vi "HP33120Aoutsine0516.VI"() -> ()   [LabVIEW 2017]
uses:
  <vilib>/Analysis/NI_AALBase.lvlib
panel:
  in  "幅值":dbl
  in  "频率":dbl
  in  "相位":dbl caption="相位（度）" format="%0.2f"
  in  "采样":i32=128
  out "波形图":waveform(dbl)(graph)
  in  "串口参数设置":enum32{"常用设置", "不常用的"}(tab)
  in  "VISA resource name":refnum<visa-resource-name>="COM1" caption="端口号"
  in  "baud rate":u32=9600 caption="波特率"
  in  "parity":u16(ring) caption="奇偶校验" items=["None", "Odd", "Even", "Mark", "Space"]
  in  "stop bits":u16(ring)=10 caption="停止位" items=["1.0"=10, "1.5"=15, "2.0"=20]
  in  "data bits":u16=8 caption="数据位" min=5 max=8 step=1
  in  "flow control":u16(ring) caption="流量控制" items=["None"=0, "XON/XOFF"=1, "RTS/CTS"=2, "DTR/DSR"=4]
  in  "termination char\n(0xA = '\\n' = LF)":u8=10 caption="EOL字串-LF" format="%.0x"
  in  "Input buffer size":u32=4096 caption="输入缓冲区大小"
  in  "XOFF Character":u8=19 format="%.0x"
  in  "XON Character":u8=17 format="%.0x"
  in  "timeout (ms)":u32=10000
  # "输出波形信息"
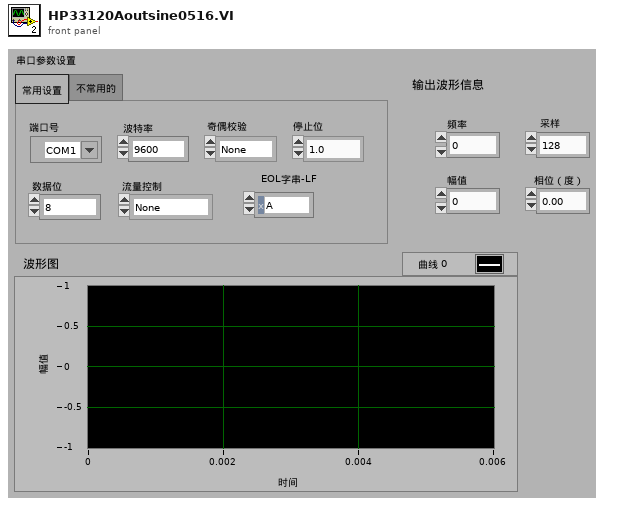
[diagram p1: front panel]
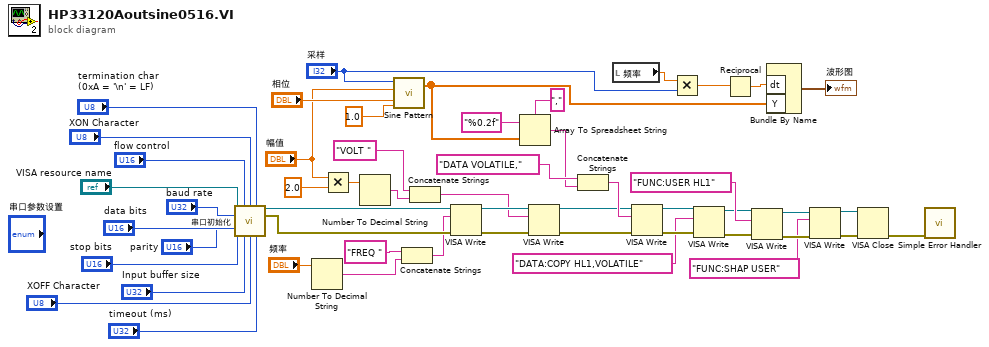
[diagram p0: block diagram]
diagram:
  n1 = call "串口初始化.vi"("VISA resource name"="VISA resource name", "flow control"="flow control", "XON Character"="XON Character", "termination char\n(0xA = '\\n' = LF)"="termination char\n(0xA = '\\n' = LF)", "baud rate"="baud rate", "data bits"="data bits", "parity"="parity", "stop bits"="stop bits", "Input buffer size"="Input buffer size", "XOFF Character"="XOFF Character", "timeout (ms)"="timeout (ms)") -> ("VISA resource name out"=w37:refnum<visa-resource-name>, "错误输出"=w36:errorcluster)  [unwired: 3 in]
  n2 = Number To Decimal String(number="频率") -> (decimal integer string=w17:string)  [unwired: 1 in]
  n3 = Multiply(x="幅值", y=2.0) -> (x*y=w1:dbl)
  n4 = Number To Decimal String(number=w1) -> (decimal integer string=w14:string)  [unwired: 1 in]
  n5 = call <vilib>:"Sine Pattern.vi"("cycles"=1.0, "phase(degrees)"="相位", "amplitude"="幅值", "samples"="采样") -> ("Sinusoidal Pattern"=w10:dbl[])  [unwired: 1 out]
  n6 = Concatenate Strings("FREQ " ("写入缓冲区"), w17) -> (w16:string)
  n7 = Concatenate Strings("VOLT " ("写入缓冲区"), w14) -> (w5:string)
  n8 = VISA Write(VISA resource name=w37, write buffer=w16, error in (no error)=w36) -> (VISA resource name out=w35:refnum<visa-resource-name>, error out=w34:errorcluster)  [unwired: 1 out]
  n9 = Array To Spreadsheet String(delimiter (Tab)="," ("分隔符(Tab)"), array=w10, 3:"%0.2f" ("格式字符串")) -> (spreadsheet string=w19:string)
  n10 = VISA Write(VISA resource name=w35, write buffer=w5, error in (no error)=w34) -> (VISA resource name out=w33:refnum<visa-resource-name>, error out=w32:errorcluster)  [unwired: 1 out]
  n11 = Concatenate Strings("DATA VOLATILE," ("写入缓冲区"), w19) -> (w38:string)
  n12 = local read "频率"() -> (w9:dbl)
  n13 = VISA Write(VISA resource name=w33, write buffer=w38, error in (no error)=w32) -> (VISA resource name out=w22:refnum<visa-resource-name>, error out=w21:errorcluster)  [unwired: 1 out]
  n14 = Multiply(x=w9, y="采样") -> (x*y=w6:dbl)
  n15 = VISA Write(VISA resource name=w22, write buffer="DATA:COPY HL1,VOLATILE" ("写入缓冲区"), error in (no error)=w21) -> (VISA resource name out=w30:refnum<visa-resource-name>, error out=w29:errorcluster)  [unwired: 1 out]
  n16 = Reciprocal(x=w6) -> (1/x=w8:dbl)
  n17 = VISA Write(VISA resource name=w30, write buffer="FUNC:USER HL1" ("写入缓冲区"), error in (no error)=w29) -> (VISA resource name out=w28:refnum<visa-resource-name>, error out=w27:errorcluster)  [unwired: 1 out]
  n18 = Bundle By Name("dt"=w8, "Y"=w10) -> (→"波形图":waveform(dbl))  [unwired: 1 in]
  n19 = VISA Write(VISA resource name=w28, write buffer="FUNC:SHAP USER" ("写入缓冲区"), error in (no error)=w27) -> (VISA resource name out=w24:refnum<visa-resource-name>, error out=w23:errorcluster)  [unwired: 1 out]
  n20 = VISA Close(VISA resource name=w24, error in (no error)=w23) -> (error out=w25:errorcluster)
  n21 = call <vilib>:"Simple Error Handler.vi"("error in (no error)"=w25) -> ()  [unwired: 4 in, 5 out]
